vi "十六进制显示强行转正常显示.vi"(1 "十六进制输入字符串":string) -> (0 "正常显示字符串":string)   [LabVIEW 2016, in "数据传输系统-06.lvlib" / "自动更新.lvlib" / "TCP文件传输系统.lvlib" / "TCP发送文件.lvlib"]
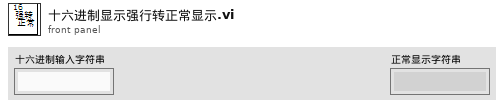
[diagram p1: front panel]
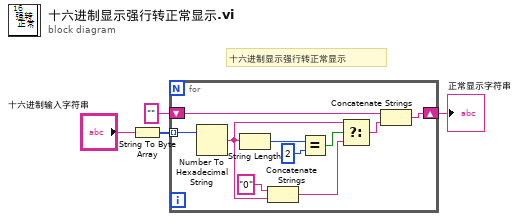
[diagram p0: block diagram]
diagram:
  # "十六进制显示强行转正常显示"
  n1 = String To Byte Array(string="十六进制输入字符串") -> (unsigned byte array=w4:u8[])
  n2 = for {
    tunnel: w4 -> [w14] mode=indexing
    shift-right: [w5] -> w1
    shift-left: "" -> [w6]
    n3 = Number To Hexadecimal String(2:w14) -> (0:w10:string)  [unwired: 1 in]
    n4 = String Length(string=w10) -> (length=w13:i32)
    n5 = Concatenate Strings("0" ("字符串"), w10) -> (w8:string)
    n6 = Equal?(x=w13, y=2) -> (x = y?=w9:bool)
    n7 = Select(t=w10, s=w9, f=w8) -> (s? t:f=w7:string)
    n8 = Concatenate Strings(w6, w7) -> (w5:string)
  }
  "正常显示字符串" <- w1
